vi "Rank.vi"(9 "DAG in":refnum<class "DAG.lvclass">) -> (4 "rank":i32[](array[numeric]))   [LabVIEW 2014, in "Raspberry Pi Compatible Compiler for LabVIEW.lvlib" / "DAG.lvclass"]
uses:
  DAG.lvclass
  DAG.lvclass/DAG.ctl
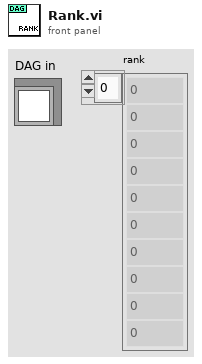
[diagram p1: front panel]
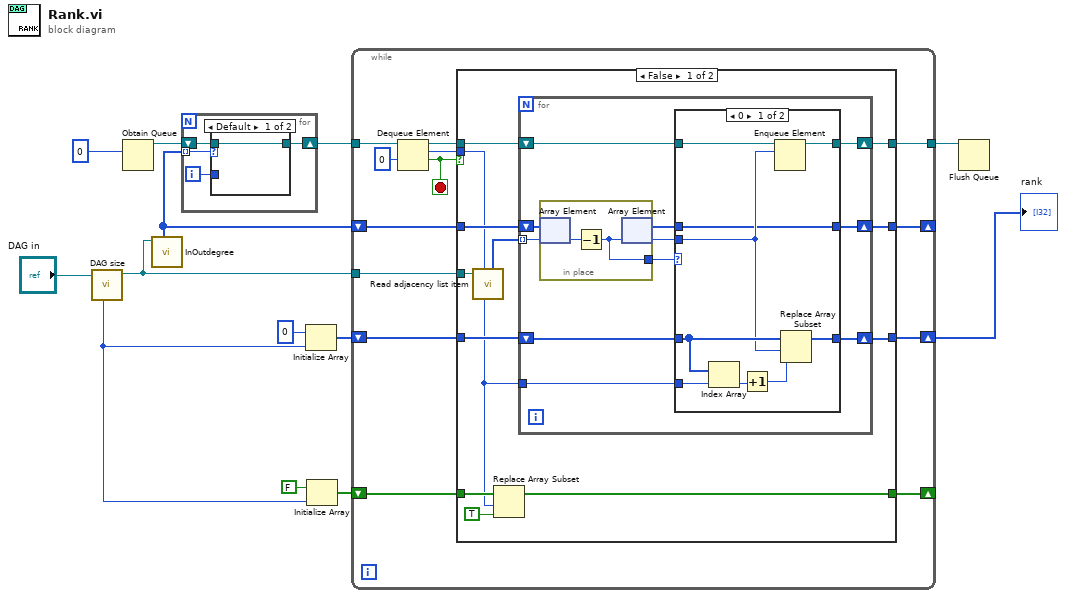
[diagram p0: block diagram]
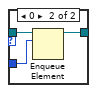
[diagram p4: hidden frame]
diagram:
  n1 = call "DAG size.vi"("DAG in"="DAG in") -> ("DAG out"=w7:refnum<class "DAG.lvclass">, "vertices"=w4:i32)  [unwired: 6 in, 1 out]
  n2 = Obtain Queue(element data type=0) -> (queue out=w10:refnum<queue>)  [unwired: 4 in, 2 out]
  n3 = call "InOutdegree.vi"("DAG in"=w7) -> ("indegree"=w6:i32[])  [unwired: 7 in, 1 out]
  n4 = for {
    tunnel: w6 -> [w15] mode=indexing
    shift-right: [w16] -> w9
    shift-left: w10 -> [w17]
    i -> [w14]
    n5 = case shown="Default" w15 {
      tunnel: w17 -> [w18 w21]
      tunnel: [w18 w20] -> w16
      tunnel: w14 -> [_ w19]
      frame Default {
      }
      frame 0 {
        n6 = Enqueue Element(queue=w21, element=w19) -> (queue out=w20:refnum<queue>)  [unwired: 2 in, 2 out]
      }
    }
  }
  n7 = Initialize Array(0, w4) -> (w8:i32[])
  n8 = Initialize Array(FALSE, w4) -> (w5:bool[])
  n9 = while {
    tunnel: w9 -> [w34]
    shift-right: [w26] -> w1
    shift-left: w8 -> [w25]
    tunnel: w7 -> [w30]
    shift-right: [w27] -> _
    shift-left: w6 -> [w28]
    shift-right: [w23] -> _
    shift-left: w5 -> [w24]
    tunnel: [w22] -> w2
    stop <- w32 stop-if-true
    n10 = Dequeue Element(queue=w34, timeout in ms (-1)=0) -> (queue out=w31:refnum<queue>, element=w29:i32, timed out?=w32:bool)  [unwired: 1 in, 1 out]
    n11 = case shown="False" w32 {
      tunnel: w31 -> [w39 w72]
      tunnel: w30 -> [w46 _]
      tunnel: w29 -> [w40 _]
      tunnel: w28 -> [w42 w75]
      tunnel: [w37 w75] -> w27
      tunnel: [w38 w74] -> w26
      tunnel: w25 -> [w41 w74]
      tunnel: w24 -> [w45 w73]
      tunnel: [w36 w73] -> w23
      tunnel: [w35 w72] -> w22
      frame False {
        n12 = call "Read adjacency list item.vi"("vertex"=w40, "DAG in"=w46) -> ("edge list"=w43:i32[])  [unwired: 6 in, 1 out]
        n13 = Replace Array Subset(array=w45, new element=TRUE ("new element/subarray"), index=w40) -> (w36:bool[])
        n14 = for {
          tunnel: w43 -> [w51] mode=indexing
          shift-right: [w48] -> w37
          shift-left: w42 -> [w57]
          shift-right: [w52] -> w38
          shift-left: w41 -> [w54]
          tunnel: w40 -> [w53]
          shift-right: [w47] -> w35
          shift-left: w39 -> [w49]
          n15 = in-place {
            in-place-border: [w70] -> w56
            n16 = in-place-array #1(w57, w51) -> (w71:i32)
            n17 = Decrement(x=w71) -> (x-1=w70:i32)
            n18 = in-place-array #1(w70) -> (w55:i32[], w50:i32)
          }
          n19 = case shown="0" w56 {
            tunnel: w55 -> [w59 w69]
            tunnel: w54 -> [w63 w68]
            tunnel: w53 -> [w66 _]
            tunnel: [w62 w68] -> w52
            tunnel: w50 -> [w60 _]
            tunnel: w49 -> [w61 w67]
            tunnel: [w59 w69] -> w48
            tunnel: [w58 w67] -> w47
            frame 0 {
              n20 = Index Array(array=w63, index=w66) -> (element=w65:i32)
              n21 = Increment(x=w65) -> (x+1=w64:i32)
              n22 = Enqueue Element(queue=w61, element=w60) -> (queue out=w58:refnum<queue>)  [unwired: 2 in, 2 out]
              n23 = Replace Array Subset(array=w63, new element=w64, index=w60) -> (w62:i32[])
            }
            frame Default {
            }
          }
        }
      }
      frame True {
      }
    }
  }
  "rank" <- w1
  n24 = Flush Queue(queue=w2) -> ()  [unwired: 1 in, 3 out]
